vi "Notes to ITX.vi"(1 "Notes":string) -> (0 "ITX Notes":string)   [LabVIEW 2019, in "LV-Data.ITX.lvclass"]
uses:
  LV-Data.ITX.lvclass
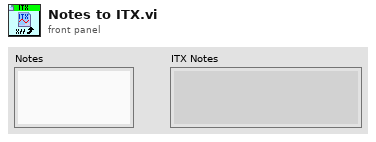
[diagram p1: front panel]
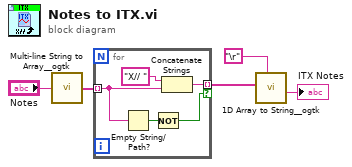
[diagram p0: block diagram]
diagram:
  n1 = call <userlib>:"Multi-line String to Array__ogtk.vi"("string"="Notes") -> ("lines"=w1:string[])
  n2 = for {
    tunnel: w1 -> [w7] mode=indexing
    tunnel: [w9] -> w3 mode=indexing if=w6
    n3 = Empty String/Path?(string/path=w7) -> (empty?=w8:bool)
    n4 = Not(x=w8) -> (.not. x?=w6:bool)
    n5 = Concatenate Strings("X// " ("string"), w7) -> (w9:string)
  }
  n6 = call <userlib>:"1D Array to String__ogtk.vi"("delimiter (Tab)"="\r", "Array of Strings"=w3) -> ("delimited string"=→"ITX Notes":string)  [unwired: 9 in]
